vi "Create Test Pattern.vi"() -> ()   [LabVIEW 2016]
uses:
  Lockin Parameters.ctl
  <vilib>/Analysis/NI_AALBase.lvlib
panel:
  in  "samples":i32=10000
  in  "Lockin parameters":T1={"Frequency"=1000000.0, "Phase"=0.0, "Syncronous"=TRUE, "Points per sine wave"=100, "DDS"=FALSE, "Frequency word"=0, "Phase word"=0, "DDS modulus"=15120, "DDS clock"=100000000.0} {"DDS clock" format="%_17pHz"; "DDS modulus" format="0x%x (%d)"; "Phase" format="%#_gdeg"; "Frequency" format="%_17pHz"}
  out "Waveform Graph":waveform(dbl)(graph)
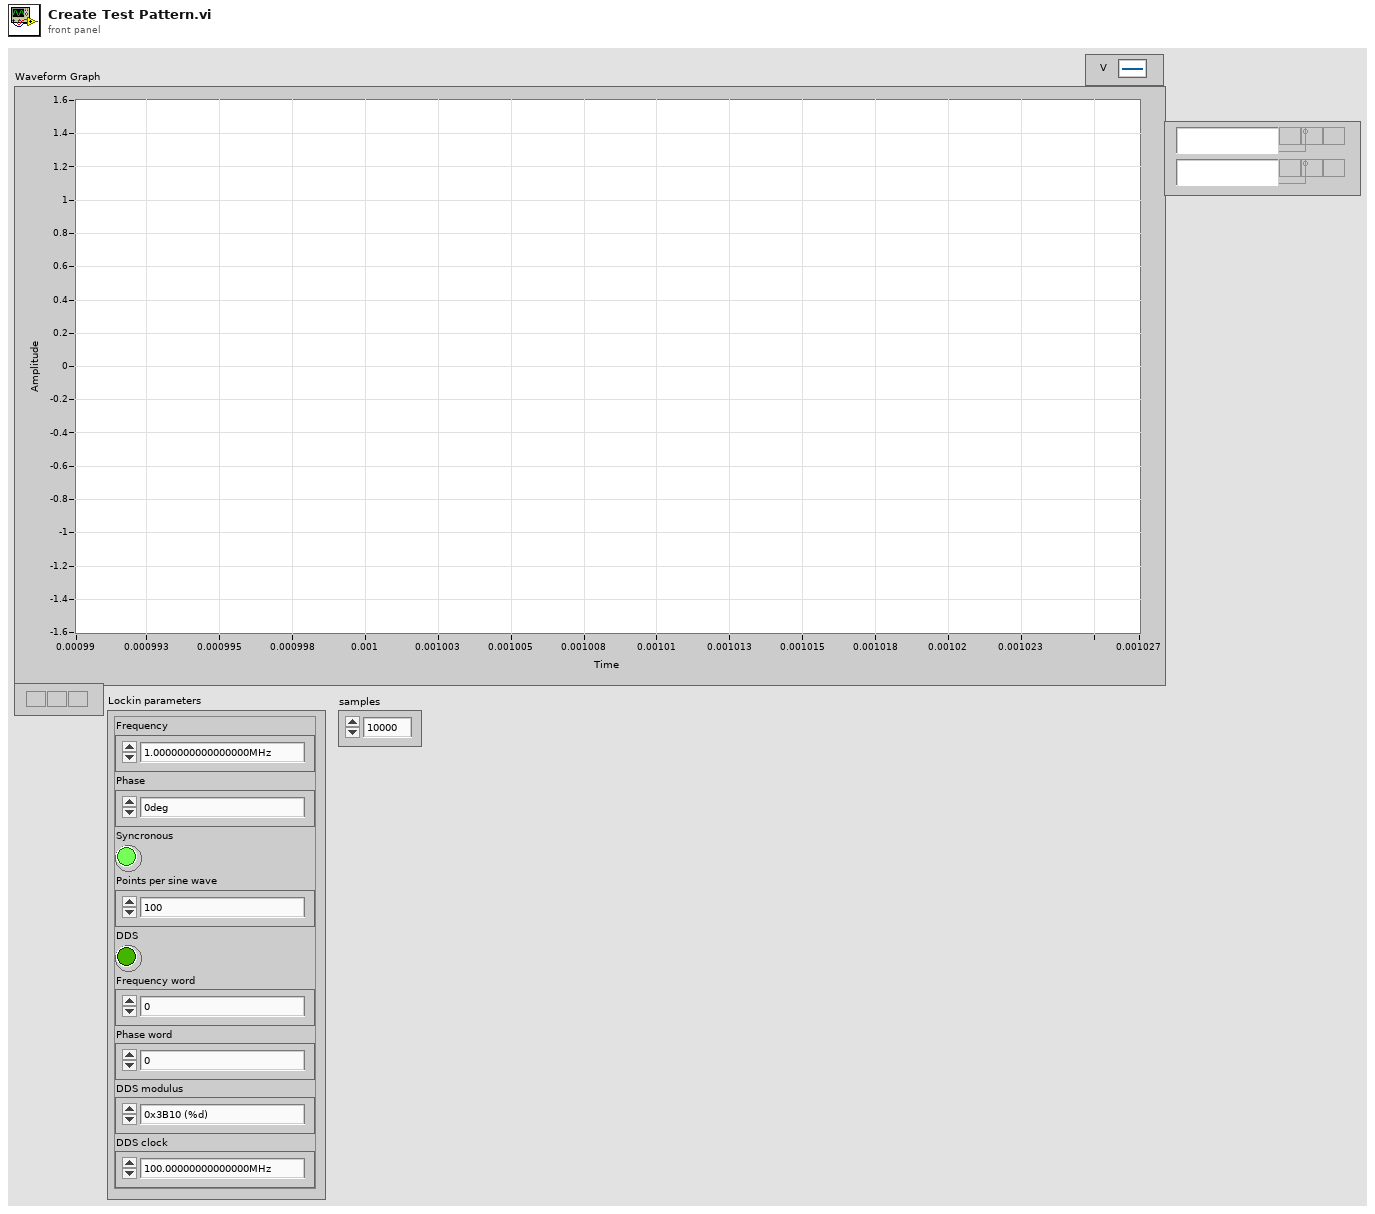
[diagram p1: front panel]
types:
  T1 = typedef "Lockin Parameters.ctl" = cluster{"Frequency":dbl, "Phase":dbl, "Syncronous":bool, "Points per sine wave":i32, "DDS":bool, "Frequency word":u32, "Phase word":u32, "DDS modulus":i64, "DDS clock":dbl}
  T2 = enum16{"open", "open or create", "create or replace", "create", "open (read-only)"}
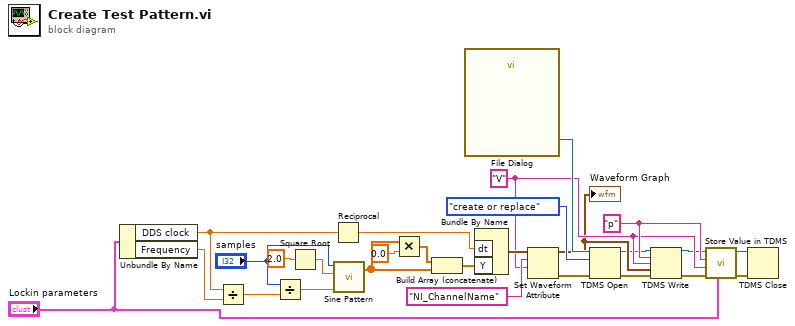
[diagram p0: block diagram]
diagram:
  w17 = "p" ("group name")
  w16 = "V" ("name")
  n1 = Unbundle By Name("Lockin parameters") -> ("DDS clock"=w5:dbl, "Frequency"=w4:dbl)
  n2 = Divide(x=w5, y=w4) -> (x/y=w2:dbl)
  n3 = Divide(x="samples", y=w2) -> (x/y=w1:dbl)
  n4 = Square Root(x=2.0) -> (sqrt(x)=w26:dbl)
  n5 = Reciprocal(x=w5) -> (1/x=w6:dbl)
  n6 = call <vilib>:"Sine Pattern.vi"("cycles"=w1, "amplitude"=w26, "samples"="samples") -> ("Sinusoidal Pattern"=w25:dbl[])  [unwired: 1 in, 1 out]
  n7 = Multiply(x=w25, y=0.0 ("cycles")) -> (x*y=w23:dbl[])
  n8 = Build Array (concatenate)(w23, w25) -> (w22:dbl[])
  n9 = call "File Dialog"() -> ("selected path"=w19:path)  [unwired: 12 in, 3 out]
  n10 = Bundle By Name("dt"=w6, "Y"=w22) -> (w21:waveform(dbl))  [unwired: 1 in]
  n11 = Set Waveform Attribute(5:w16, 6:"NI_ChannelName" ("name"), 7:w21) -> (0:w13:errorcluster, 3:w15:waveform(dbl))  [unwired: 1 in, 1 out]
  "Waveform Graph" <- w15
  n12 = TDMS Open(8:w13, 10:T2."create or replace" ("operation (0:open)"), 11:w19) -> (0:w14:errorcluster, 3:w10:refnum<k34>)  [unwired: 4 in]
  n13 = TDMS Write(0:w10, 5:w17, 7:w16, 9:w15, 11:w14) -> (4:w11:refnum<k34>, 15:w12:errorcluster)  [unwired: 1 in, 2 out]
  n14 = call "Store Value in TDMS.vi"("Value"="Lockin parameters", "Error In"=w12, "channel name"=w16, "group name"=w17, "tdms file"=w11) -> ("Error Out"=w9:errorcluster, "tdms file out"=w8:refnum<k34>)  [unwired: 3 in, 2 out]
  n15 = TDMS Close(8:w9, 11:w8) -> ()  [unwired: 2 out]
